vi "program seq..vi"(6 "IOList":T3, 7 "Cluster data":T5, 11 "Filepath":path=path "E:/My Project/2018-2019/Under development/Minda Ind. Switch -ID 144-145/Project/data/trail pro -12.txt") -> (0 "Error Out":errorcluster)   [LabVIEW 2015]
uses:
  Control PB/Active.ctl
  Control PB/deactive.ctl
  Control PB/output control.ctl
  Control PB/input control.ctl
  Control PB/timer.ctl
  Control PB/Remove list.ctl
  Control Button/Exit.ctl
  Control PB/Add_s.ctl
  Control PB/Delete_.ctl
  Control Button/Save.ctl
  Control PB/motor.ctl
  Control PB/Camera.ctl
  Control PB/Barcode.ctl
  Galobal variable_TI.vi
panel:
  out "Step List 5":string[](array[string])
  in  "CAN":bool
  in  "Feature Step edit":bool
  out "Step List 4":string[](array[string])
  out "Step List 3":string[](array[string])
  in  "Barcode":T1
  in  "Camera":T2
  out "x <= y?":bool
  out "Cancel":bool
  out "Step List 2":string[](array[string])
  out "Pokayoka Result":cluster{"Sensor Name":string, "Boolean":bool}[](array[cluster])
  in  "Feed Back Channel":i32[](listbox)=[0]
  out "Input":bool[](array[boolean])
  out "Feature List (Out) 2":T4(array[cluster])
  out "error out 2":errorcluster
  in  "Control":bool
  out "Station No":string
  out "Model Name":string
  out "Model":string
  in  "Motor":T6
  in  "Feature List":i32(listbox) caption="Steps List"
  in  "Deletefeature list":T7
  in  "Add feature list":T8
  in  "Deactive":T9
  in  "Active":T10
  in  "Program step":i32(listbox)
  in  "Remove Step":T11
  in  "Wait Time":u32=100 caption="Timer(ms)" max=600000 step=1
  in  "Timer":T12
  in  "Save":T13
  in  "stop":T14
  in  "op Add":T15
  in  "Input Add":T16
  out "Step List":string[](array[string])
  out "output cluster":T17
  in  "Analog":bool
  in  "Analog Input":i32[](listbox)=[0]
  in  "Control Channel":i32[](listbox)=[7]
  in  "Steps":T18(array[cluster])
  in  "Program mode":string="Data"
  out "error out":errorcluster
  out "Feature List (Out)":T19(array[cluster])
  # "Program Sequence Window"
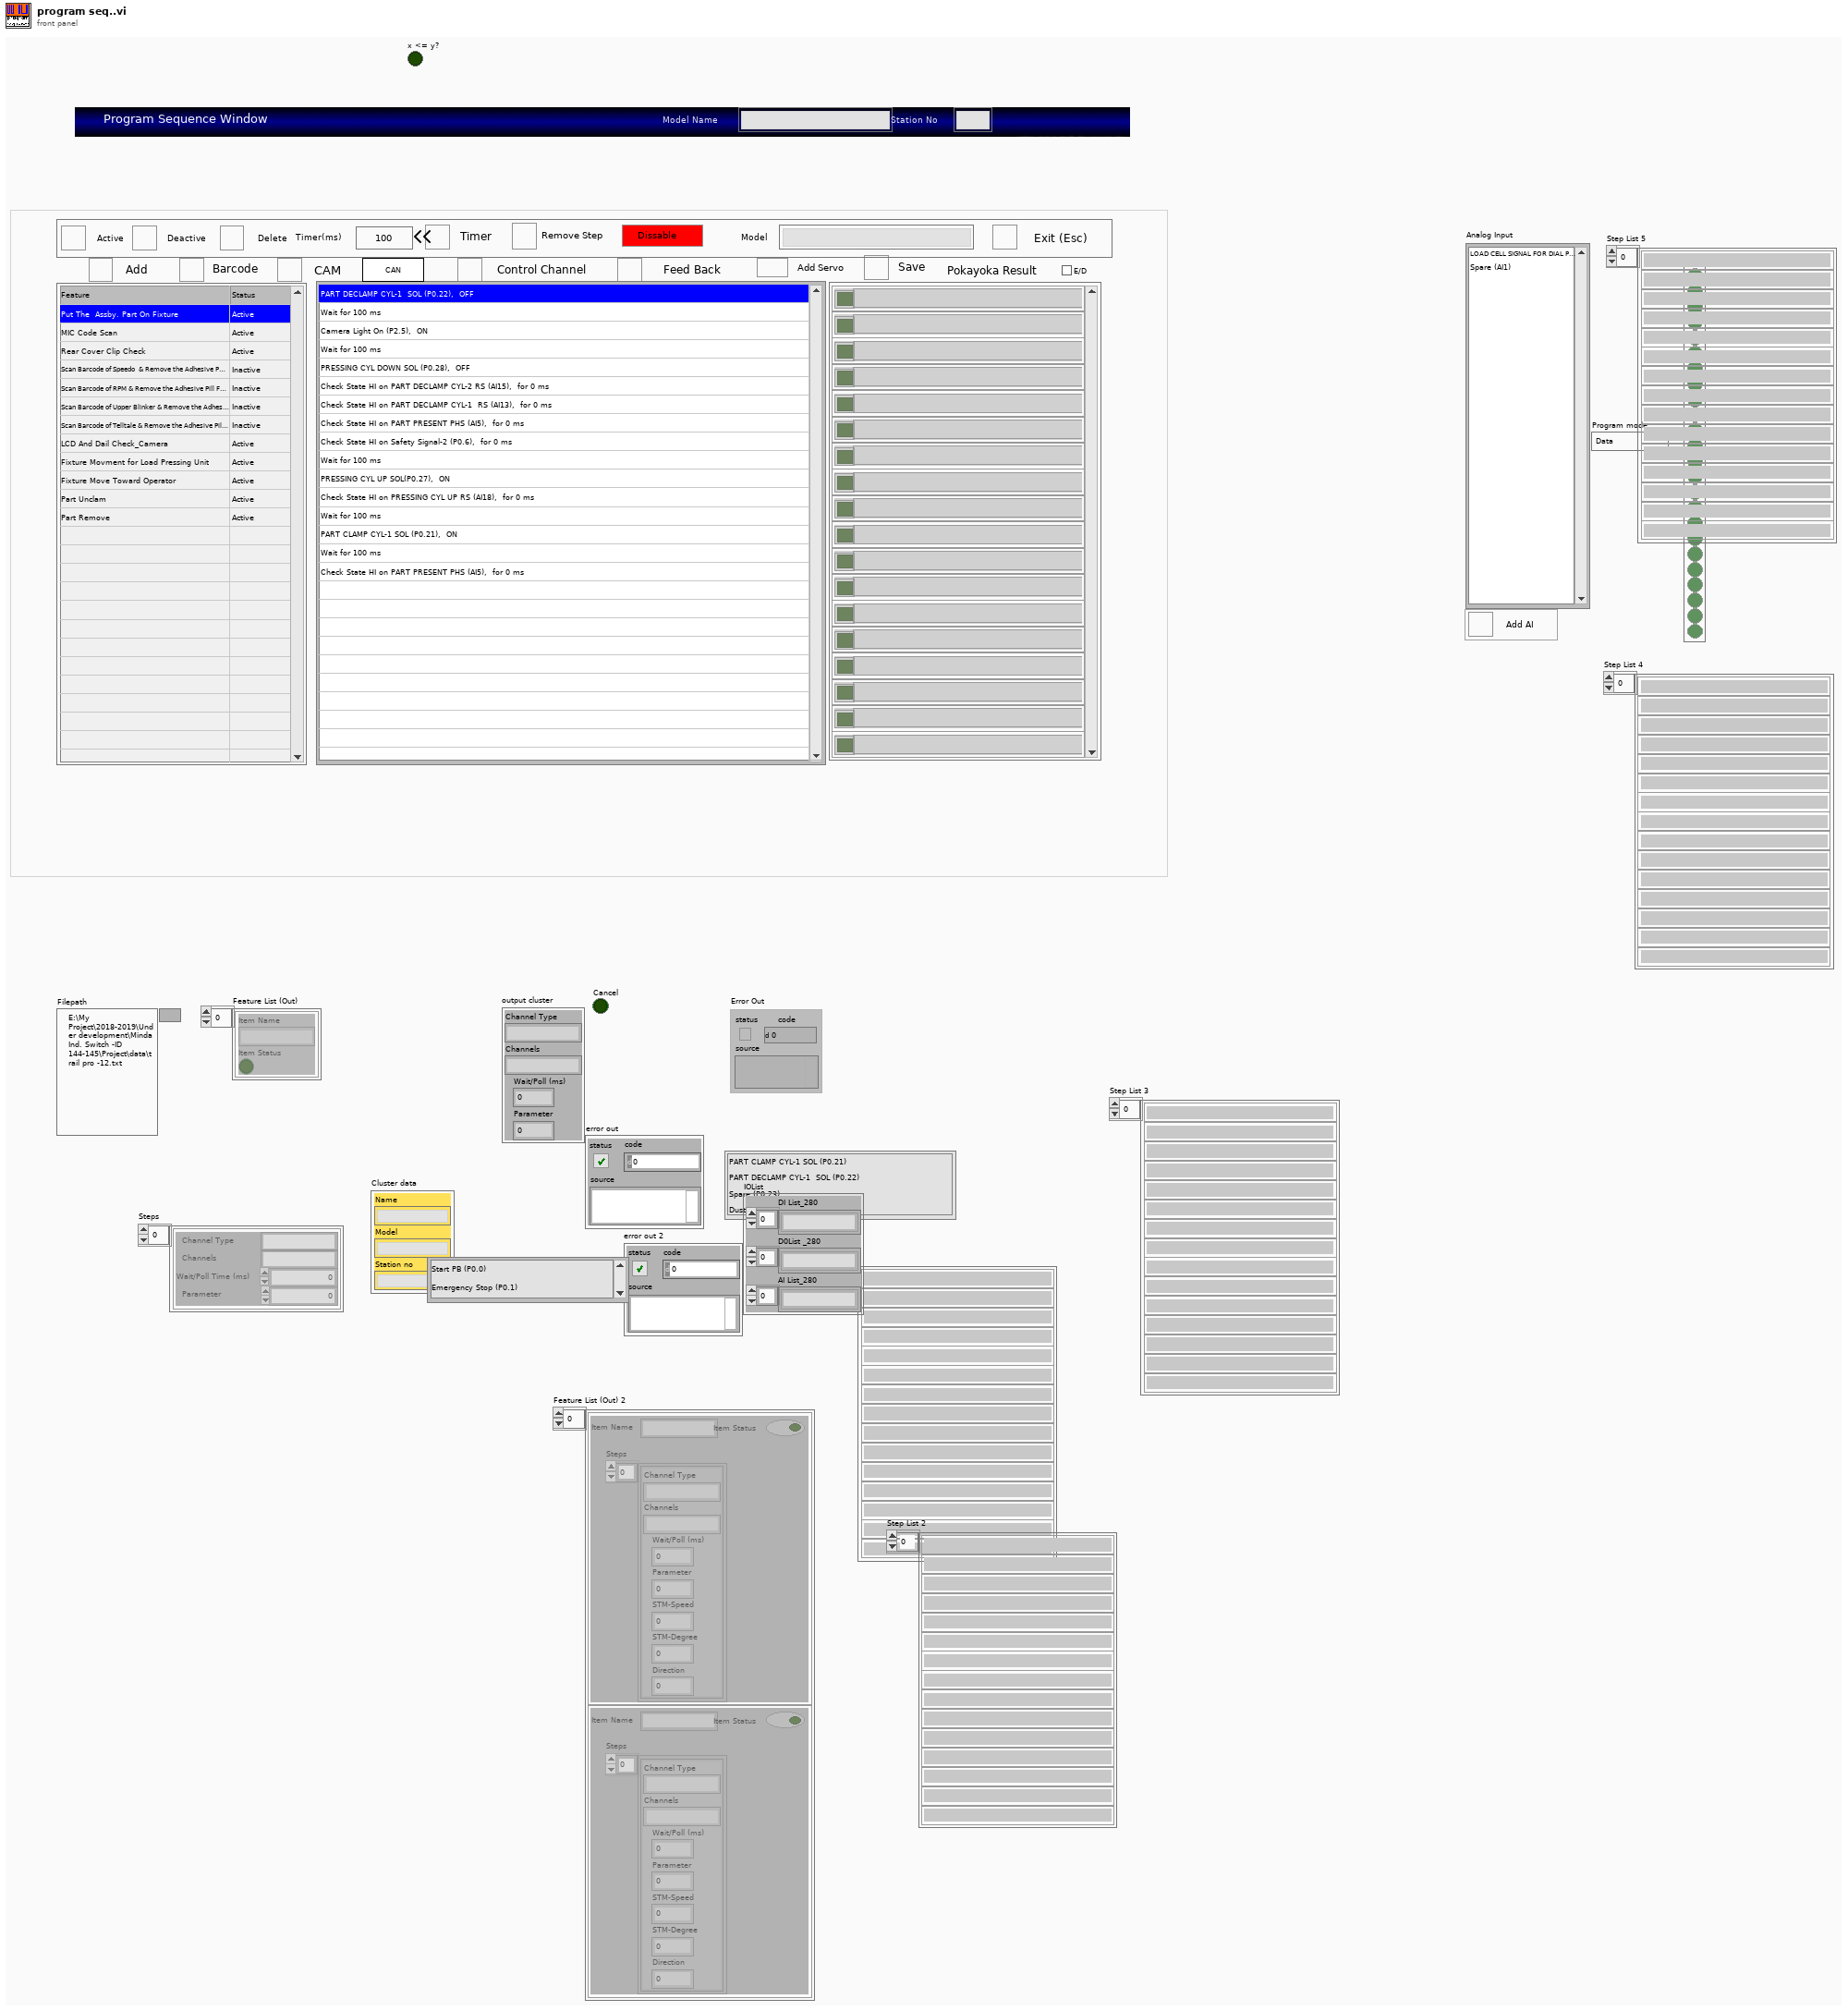
[diagram p1: front panel]
types:
  T1 = typedef "Barcode.ctl" = bool
  T2 = typedef "Camera.ctl" = bool
  T3 = cluster{"DI List_280":string[], "D0List _280":string[], "AI List_280":string[]}
  T4 = cluster{"Item Name":string, "Item Status":bool, "Steps":cluster{"Channel Type":string, "Channels":string, "Wait/Poll (ms)":u32, "Parameter":u8, "STM-Speed":i32, "STM-Degree":u32, "Direction":u8}[]}[]
  T5 = cluster{"Name":string, "Model":string, "Station no":string}
  T6 = typedef "motor.ctl" = bool
  T7 = typedef "Delete_.ctl" = bool
  T8 = typedef "Add_s.ctl" = bool
  T9 = typedef "deactive.ctl" = bool
  T10 = typedef "Active.ctl" = bool
  T11 = typedef "Remove list.ctl" = bool
  T12 = typedef "timer.ctl" = bool
  T13 = typedef "Save.ctl" = bool
  T14 = typedef "Exit.ctl" = bool
  T15 = typedef "output control.ctl" = bool
  T16 = typedef "input control.ctl" = bool
  T17 = cluster{"Channel Type":string, "Channels":string, "Wait/Poll (ms)":u32, "Parameter":u8}
  T18 = cluster{"Channel Type":string, "Channels":string, "Wait/Poll Time (ms)":u32, "Parameter":u8}[]
  T19 = cluster{"Item Name":string, "Item Status":bool}[]
  T20 = cluster{"Channel Type":string, "Channels":string, "Wait/Poll (ms)":u32, "Parameter":u8, "STM-Speed":i32, "STM-Degree":i32, "Direction":u8}
  T21 = cluster{"Item Name":string, "Item Status":bool, "Steps":cluster{"Channel Type":string, "Channels":string, "Wait/Poll (ms)":u32, "Parameter":u8, "STM-Speed":i32, "STM-Degree":u32, "Direction":u8}[]}
  T22 = cluster{"Channel Type":string, "Channels":string, "Wait/Poll (ms)":u32, "Parameter":u8, "STM-Speed":i32, "STM-Degree":u32, "Direction":u8}[]
  T23 = typedef "CAN.ctl" = enum16{"TFT/LCD Power On", "TFT/LCD Power Off", "KM CHeck"}
  T24 = cluster{"Item Name":string, "Active":T10, "Steps":cluster{"Channel Type":string, "Channels":string, "Wait/Poll (ms)":u32, "Parameter":u8, "STM-Speed":i32, "STM-Degree":u32, "Direction":u8}[]}
  T25 = cluster{"Channel Type":string, "Channels":string, "Wait/Poll (ms)":u32, "Parameter":u8, "STM-Speed":i32, "STM-Degree":i32, "Direction":u8}[]
  T26 = cluster{"Feature name ":string, bool, cluster{"Channel Type":string, "Channels":string, "Wait/Poll (ms)":u32, "Parameter":u8, "STM-Speed":i32, "STM-Degree":i32, "Direction":u8}[]}
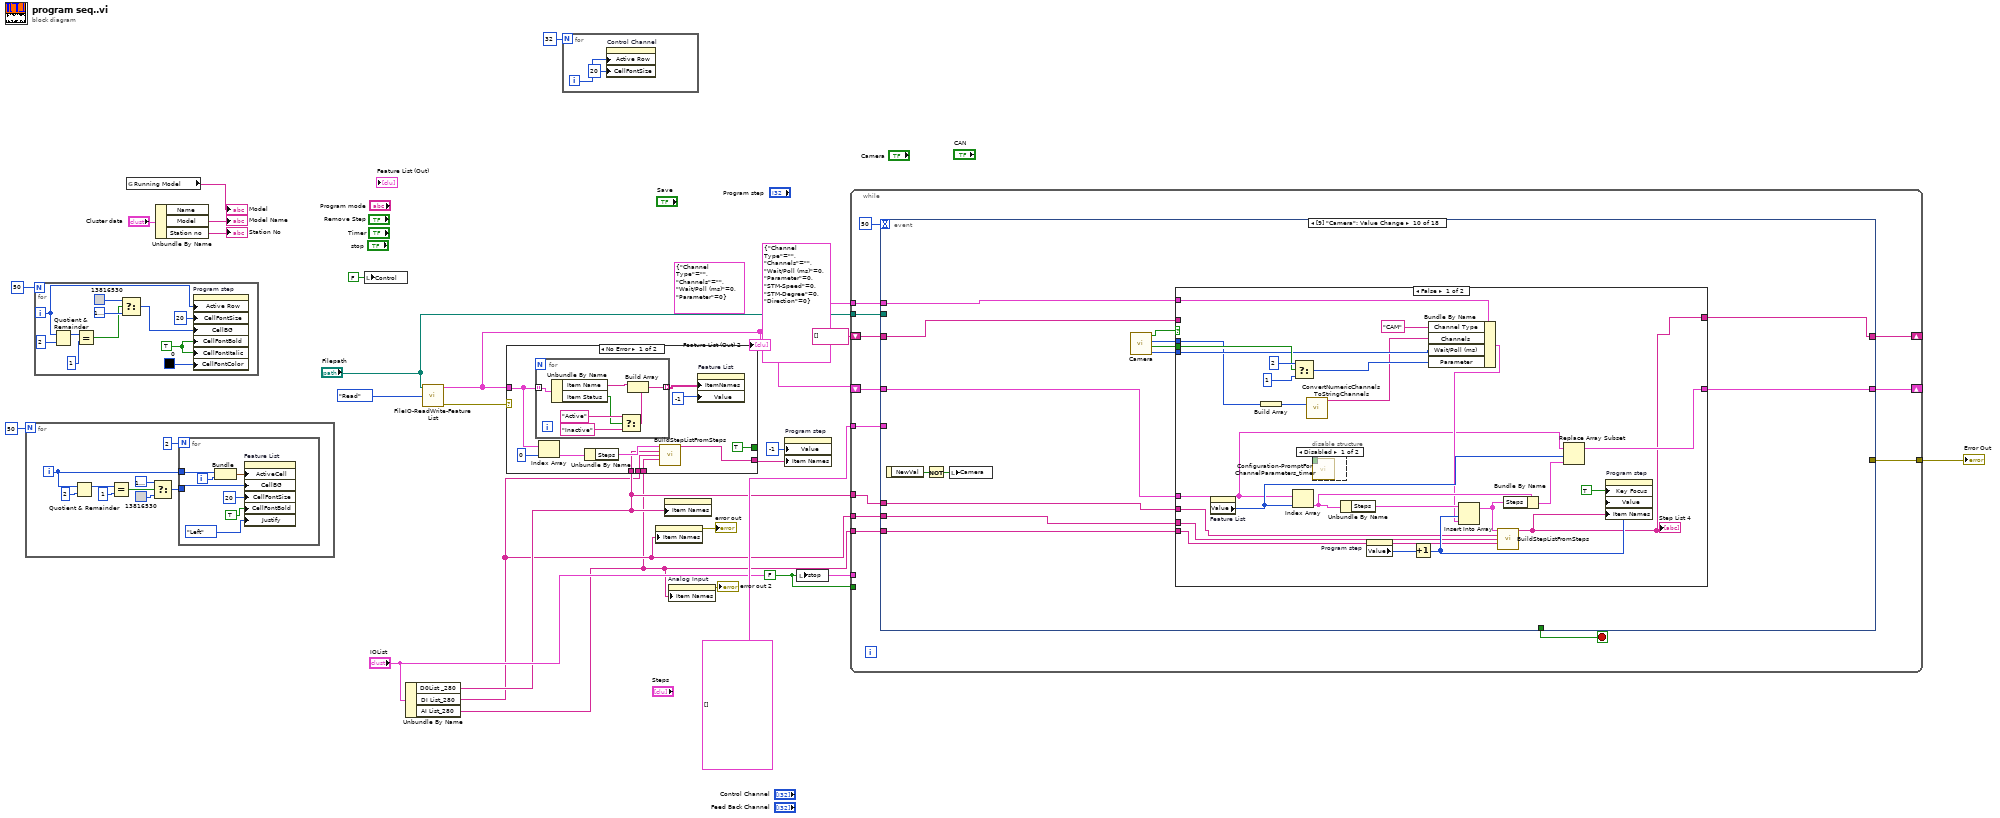
[diagram p0: block diagram]
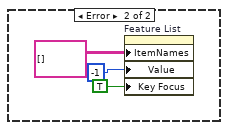
[diagram p2: hidden frame]
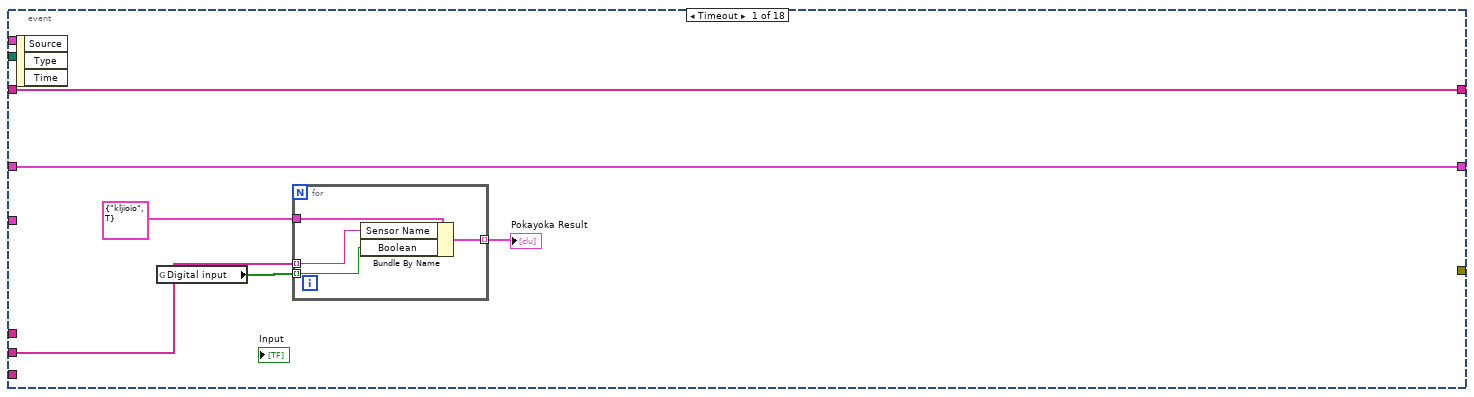
[diagram p3: hidden frame]
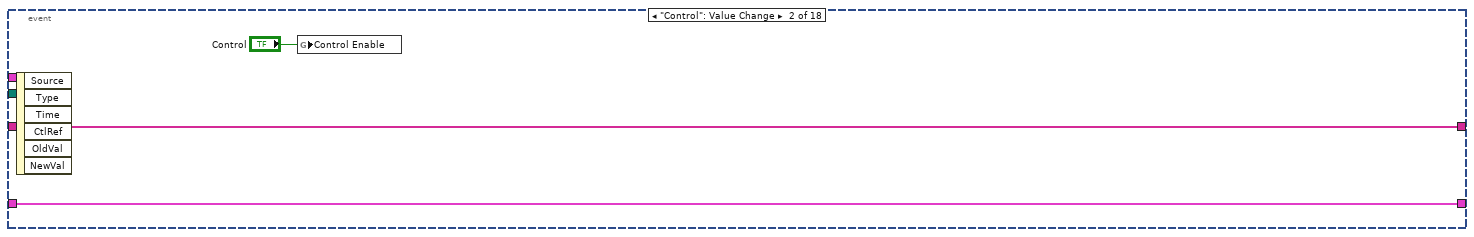
[diagram p4: hidden frame]
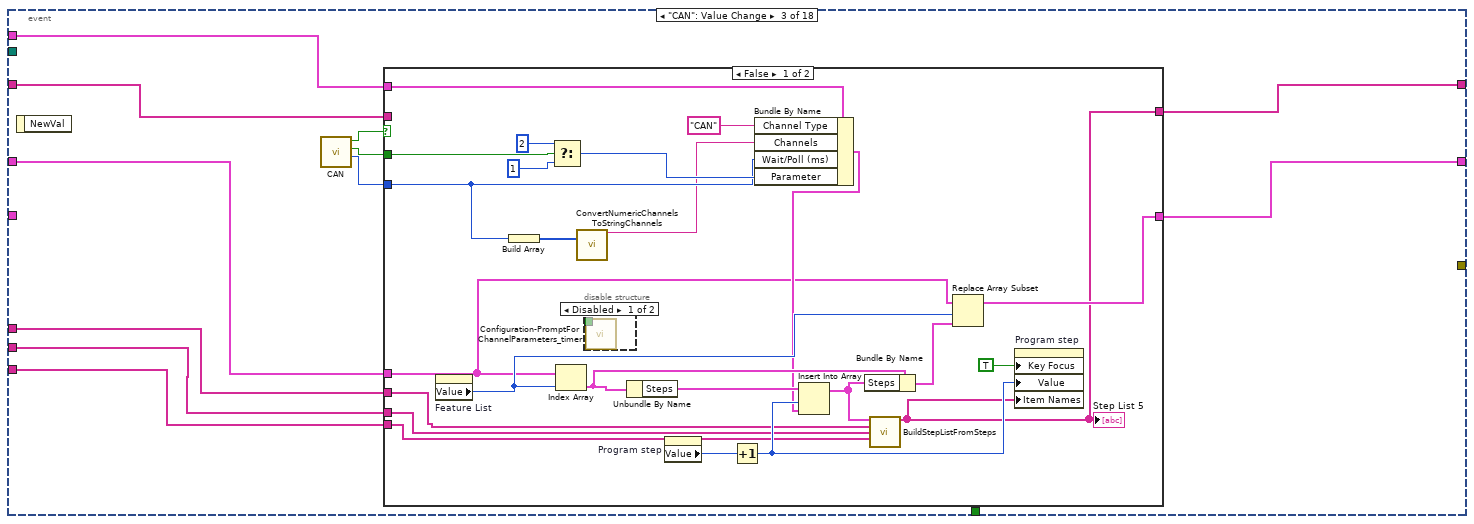
[diagram p5: hidden frame]
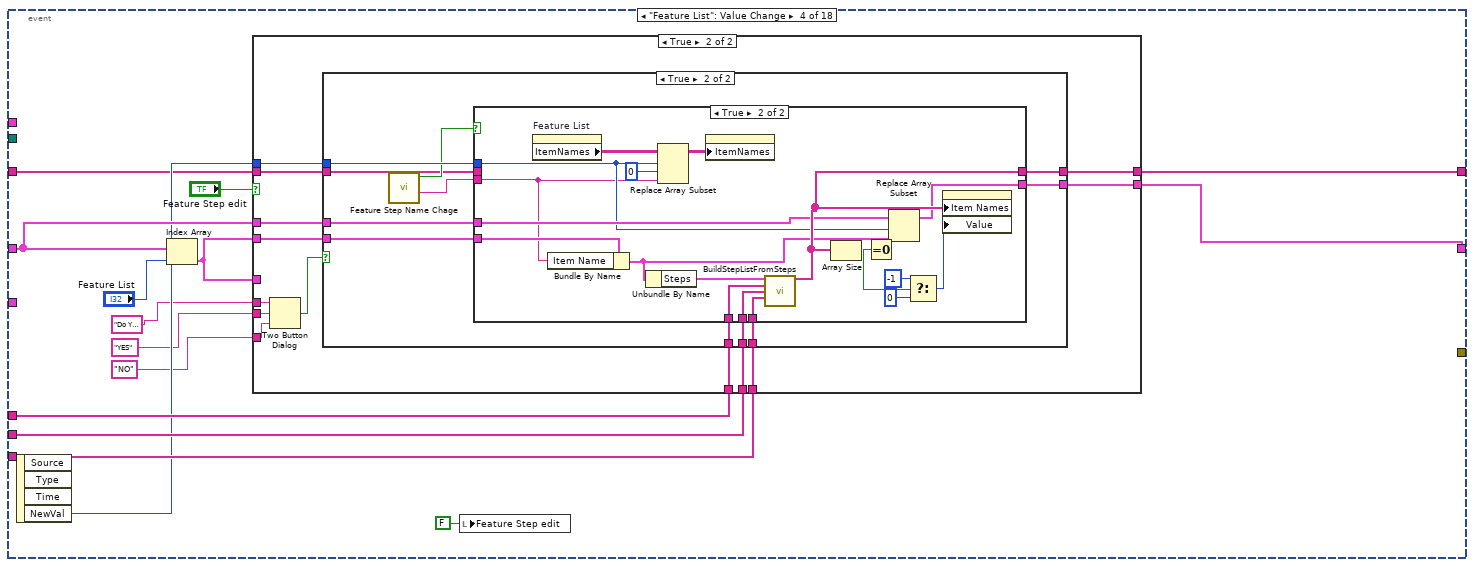
[diagram p8: hidden frame]
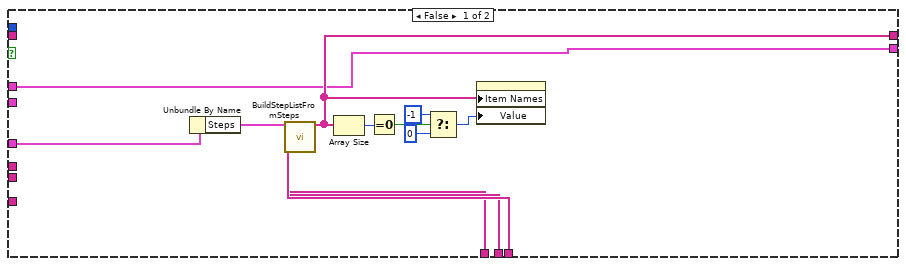
[diagram p9: hidden frame]
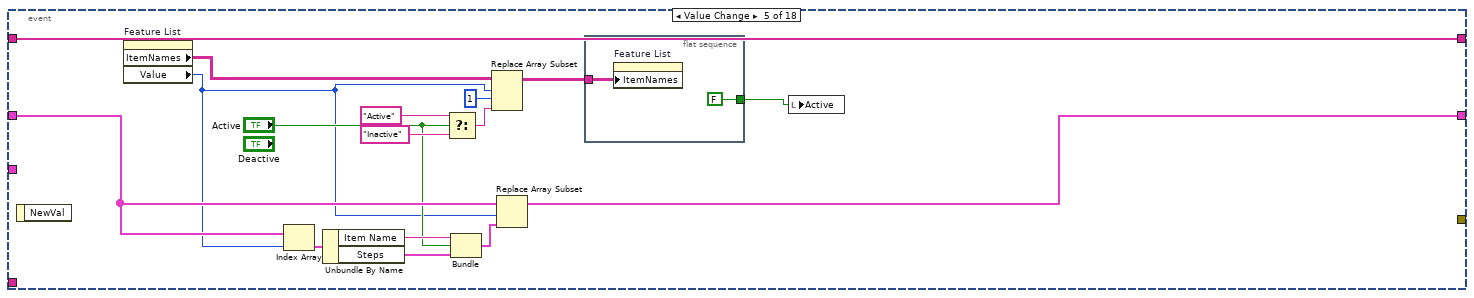
[diagram p12: hidden frame]
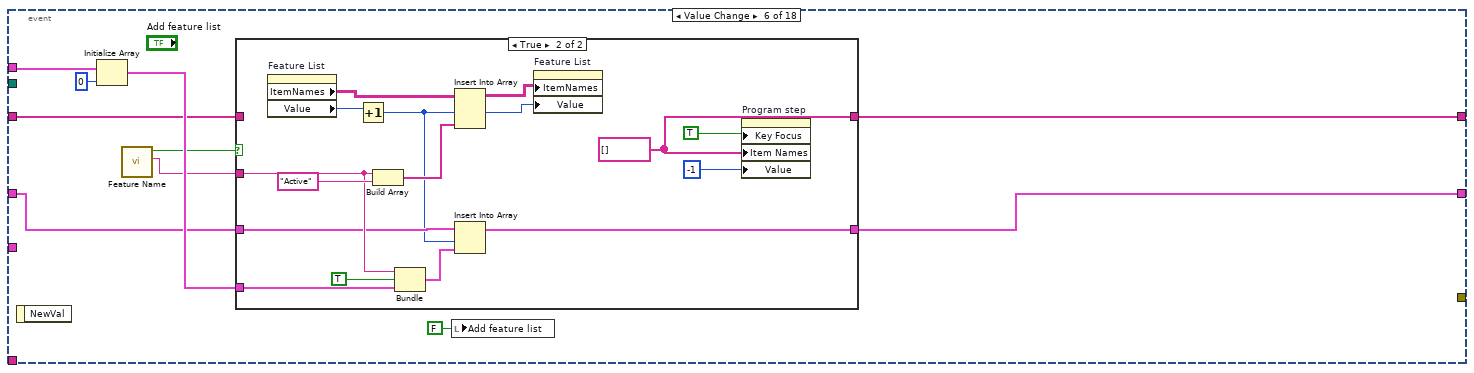
[diagram p13: hidden frame]
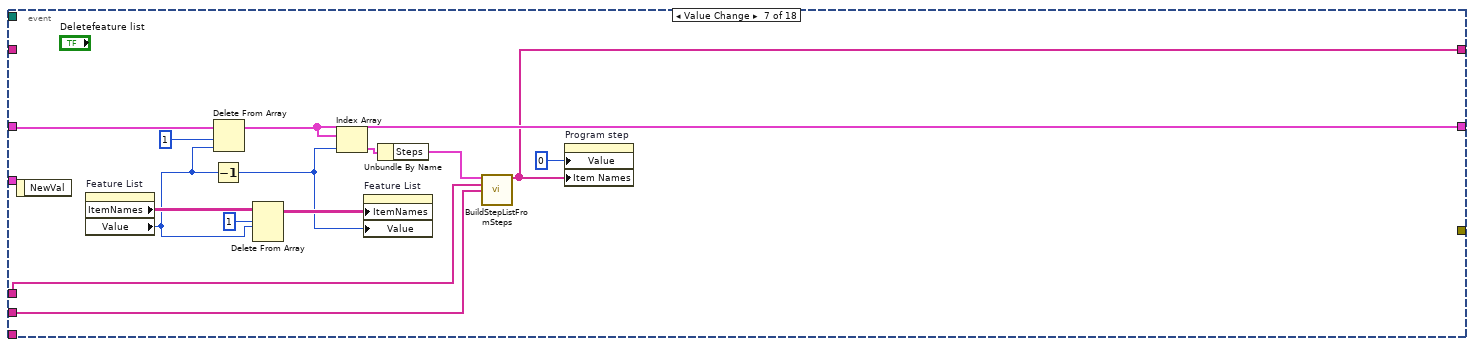
[diagram p15: hidden frame]
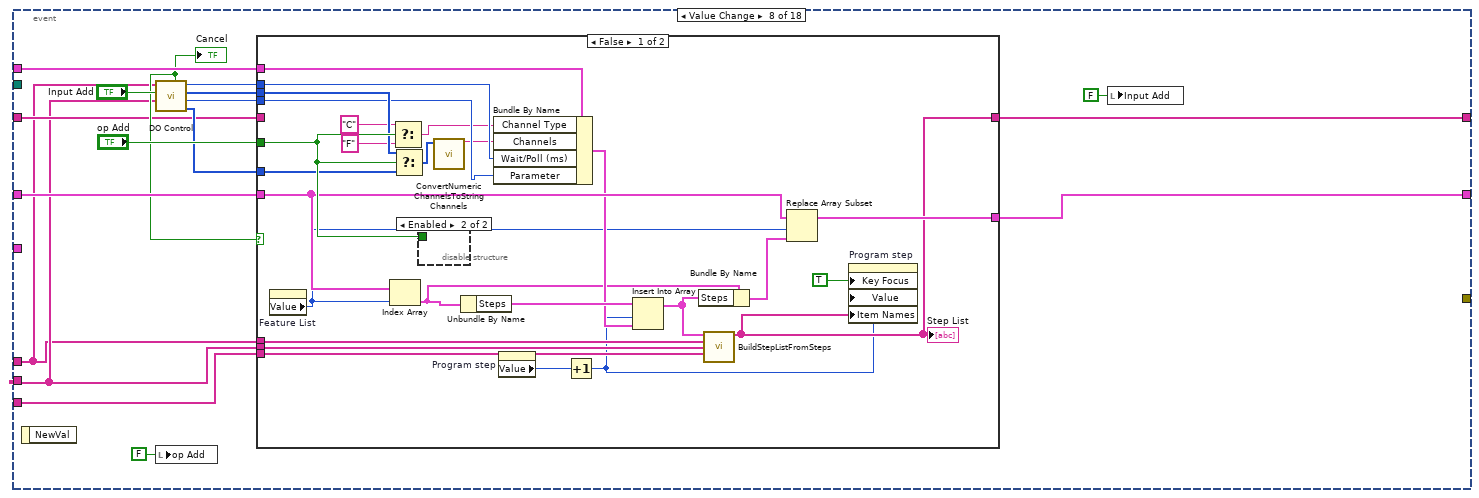
[diagram p16: hidden frame]
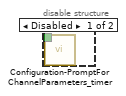
[diagram p17: hidden frame]
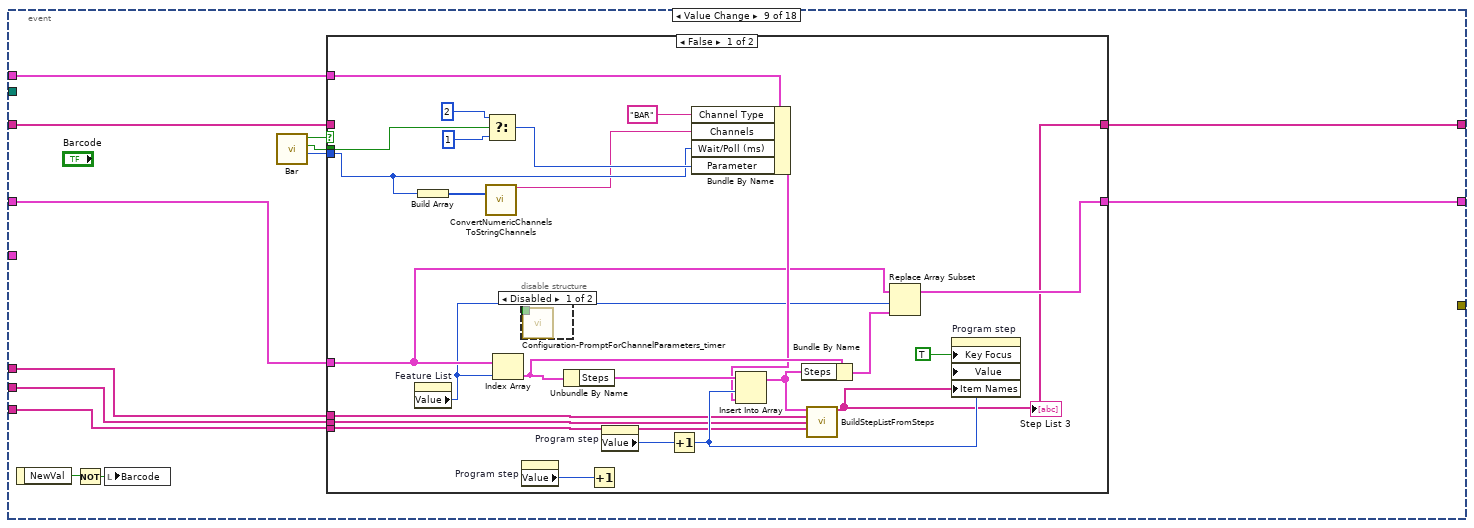
[diagram p19: hidden frame]
diagram:
  w9 = FALSE ("stop")
  (unwired) T17 {"Channel Type"="", "Channels"="", "Wait/Poll (ms)"=0, "Parameter"=0} ("Step")
  n1 = for {
    N: 50 -> [_]
    i -> [w33]
    n2 = Quotient & Remainder(x=w33, y=2) -> (x-y*floor(x/y)=w31:i32)  [unwired: 1 out]
    n3 = Equal?(x=w31, y=1) -> (x = y?=w29:bool)
    n4 = Select(t=u32 16777225 ("Color Box"), s=w29, f=u32 13816530 ("Color Box")) -> (s? t:f=w26:u32)
    n5 = for {
      N: 2 -> [_]
      tunnel: w33 -> [w41]
      tunnel: w26 -> [w38]
      i -> [w40]
      n6 = Bundle(w41, w40) -> (w39:cluster{i32, i32})  [unwired: 1 in]
      n7 = property on="Feature List" class="MCListbox (strict)"("ActiveCell"=w39, "CellBG"=w38, "CellFontSize"=u32 20 ("Active Cell:Cell Font:Size"), "CellFontBold"=TRUE ("Active Cell:Cell Font:Bold"), "Justify"=enum16{"Left", "Center", "Right"}."Left" ("Active Cell:Cell Justification")) -> ()  [unwired: 2 in, 2 out]
    }
  }
  n8 = for {
    N: 50 -> [_]
    i -> [w46]
    w43 = TRUE
    n9 = Quotient & Remainder(x=w46, y=2) -> (x-y*floor(x/y)=w49:i32)  [unwired: 1 out]
    n10 = Equal?(x=w49, y=1) -> (x = y?=w47:bool)
    n11 = Select(t=u32 13816530 ("Color Box"), s=w47, f=u32 16777226 ("Color Box")) -> (s? t:f=w44:u32)
    n12 = property on="Program step" class="LstBox (strict)"("Active Row"=w46, "CellFontSize"=u32 20 ("Active Row:Cell Font:Size"), "CellBG"=w44, "CellFontBold"=w43, "CellFontItalic"=w43, "CellFontColor"=u32 0 ("Color Box")) -> ()  [unwired: 2 in, 2 out]
  }
  n13 = global read "Galobal variable_TI.vi" "Running Model"() -> (→"Model":string)
  n14 = Unbundle By Name("Cluster data") -> ("Model"=→"Model Name":string, "Station no"=→"Station No":string)  [unwired: 1 out]
  n15 = local write "Control"(FALSE ("Control")) -> ()
  n16 = Unbundle By Name("IOList") -> ("D0List _280"=w5:string[], "DI List_280"=w4:string[], "AI List_280"=w3:string[])
  n17 = call "FileIO-ReadWrite-FeatureList.vi"("Filepath"="Filepath", "Read/Write"=enum16{"Read", "Write"}."Read") -> ("Feature List (Out)"=w16:T4, "Error Out"=w20:errorcluster)  [unwired: 12 in]
  "Feature List (Out) 2" <- w16
  n18 = case shown="No Error" w20 {
    tunnel: w16 -> [w63 _]
    tunnel: w5 -> [w59 _]
    tunnel: w4 -> [w58 _]
    tunnel: w3 -> [w57 _]
    tunnel: [w56 _] -> w19
    tunnel: [TRUE ("Key Focus") _] -> _
    frame No Error {
      n19 = for {
        tunnel: w63 -> [w70] mode=indexing
        tunnel: [w64] -> w54 mode=indexing
        n20 = Unbundle By Name(w70) -> ("Item Name"=w66:string, "Item Status"=w67:bool)
        n21 = Select(t="Active", s=w67, f="Inactive") -> (s? t:f=w65:string)
        n22 = Build Array(w66, w65) -> (w64:string[])
      }
      n23 = Index Array(array=w63, index=0) -> (element=w61:T21)
      n24 = Unbundle By Name(w61) -> ("Steps"=w60:T22)
      n25 = call "BuildStepListFromSteps.vi"("Steps"=w60, "Control Channels"=w59, "Feedback Channels"=w58, "AI"=w57) -> ("Step List"=w56:string[])  [unwired: 11 in]
      n26 = property on="Feature List" class="MCListbox (strict)"("ItemNames"=w54, "Value"=-1 ("Feautre list")) -> ()  [unwired: 2 in, 2 out]
    }
    frame Error {
      n27 = property on="Feature List" class="MCListbox (strict)"("ItemNames"=string[][] [] ("Item Names"), "Value"=-1 ("Feautre list"), "Key Focus"=TRUE) -> ()  [unwired: 2 in, 2 out]
    }
  }
  n28 = for {
    N: 32 -> [_]
    i -> [w75]
    n29 = property on="Control Channel" class="LstBox (strict)"("Active Row"=w75, "CellFontSize"=u32 20 ("Active Row:Cell Font:Size")) -> ()  [unwired: 2 in, 2 out]
  }
  n30 = property on="Feed Back Channel" class="LstBox (strict)"("Item Names"=w4) -> (error out=→"error out":errorcluster)  [unwired: 2 in, 1 out]
  n31 = property on="Control Channel" class="LstBox (strict)"("Item Names"=w5) -> ()  [unwired: 2 in, 2 out]
  n32 = property on="Analog Input" class="LstBox (strict)"("Item Names"=w3) -> (error out=→"error out 2":errorcluster)  [unwired: 2 in, 1 out]
  n33 = property on="Program step" class="LstBox (strict)"("Value"=-1 ("Step feautre list"), "Item Names"=w19) -> ()  [unwired: 2 in, 2 out]
  n34 = local write "stop"(w9) -> ()
  n35 = while {
    shift-right: [w86] -> _
    shift-left: w16 -> [w77]
    tunnel: T20 {"Channel Type"="", "Channels"="", "Wait/Poll (ms)"=0, "Parameter"=0, "STM-Speed"=0, "STM-Degree"=0, "Direction"=0} ("Step") -> [w87]
    shift-right: [w85] -> _
    shift-left: string[] [] ("Step List") -> [w84]
    tunnel: w5 -> [w83]
    tunnel: w4 -> [w82]
    tunnel: [w81] -> w23
    tunnel: w3 -> [w80]
    tunnel: T4 [] ("Feature List (Out) 2") -> [w79]
    tunnel: "Filepath" -> [w78]
    tunnel: w9 -> [_]
    tunnel: "IOList" -> [_]
    stop <- w88 stop-if-true
    n36 = event shown="[9] \"Camera\": Value Change" {
      selector: _ -> [_ _ _ _ _ _ _ _ _ _ _ _ _ _ _ _ _ _]
      dyn-events: _ -> [_ _ _ _ _ _ _ _ _ _ _ _ _ _ _ _ _ _]
      timeout: 50 -> [_ _ _ _ _ _ _ _ _ _ _ _ _ _ _ _ _ _]
      tunnel: [_ _ _ _ _ _ _ _ _ _ _ _ _ _ _ TRUE ("stop") _ TRUE ("Discard?")] -> w88
      tunnel: w77 -> [w94 w100 w102 w148 w221 w238 w270 w286 w326 w369 w411 w441 w462 w484 w493 w553 w575 w652]
      tunnel: w87 -> [_ _ w109 _ _ w241 _ w289 w331 w373 w418 w446 w471 _ _ _ w576 _]
      tunnel: [w94 w100 w103 w147 w219 w237 w269 w287 w325 w368 w406 w433 w461 w483 w495 w553 w571 w652] -> w86
      tunnel: [w93 w101 w107 w154 w218 w234 w264 w285 w324 w367 w405 w432 w458 w478 w510 w552 w570 w653] -> w85
      tunnel: w84 -> [w93 w101 w108 w140 w218 w233 _ w276 w319 w363 _ _ _ _ _ w552 w569 w653]
      tunnel: w83 -> [_ _ w112 w153 _ _ w266 w274 w327 w370 w408 w438 w460 w480 w512 _ w572 _]
      tunnel: w82 -> [w92 _ w111 w152 _ _ w265 w275 w328 w371 w409 w437 w459 w479 w511 _ w573 _]
      tunnel: [_ _ _ _ _ _ _ _ _ _ _ _ _ _ w503 _ _ _] -> w81
      tunnel: w80 -> [_ _ w110 w151 _ _ _ w284 w329 w372 w410 w436 w457 _ w504 _ w574 _]
      tunnel: w79 -> [_ _ _ _ _ _ _ _ _ _ _ _ _ _ w509 _ _ _]
      tunnel: w78 -> [_ _ _ _ _ _ _ _ _ _ _ _ _ _ w494 _ _ _]
      event Timeout {
        n37 = event-data() -> ()  [unwired: 1 in, 3 out]
        n38 = global read "Galobal variable_TI.vi" "Digital input"() -> (w89:bool[])
        n39 = for {
          tunnel: w92 -> [w97] mode=indexing
          tunnel: cluster{"Sensor Name":string, "Boolean":bool} {"Sensor Name"="kljioio", "Boolean"=TRUE} ("Cluster") -> [w98]
          tunnel: [w96] -> w90 mode=indexing
          tunnel: w89 -> [w95] mode=indexing
          n40 = Bundle By Name(cluster=w98, "Sensor Name"=w97, "Boolean"=w95) -> (w96:cluster{"Sensor Name":string, "Boolean":bool})
        }
        "Pokayoka Result" <- w90
      }
      event "Control": Value Change {
        n41 = event-data() -> ()  [unwired: 1 in, 6 out]
        n42 = global write "Galobal variable_TI.vi" "Control Enable"("Control") -> ()
      }
      event "CAN": Value Change {
        n43 = event-data() -> ()  [unwired: 1 in, 1 out]
        n44 = call "CAN.vi"() -> ("CAN Sele"=w106:T23, "CAN"=w105:bool, "Out"=w104:bool)  [unwired: 9 in]
        n45 = case shown="False" w104 {
          tunnel: w110 -> [w123 _]
          tunnel: w111 -> [w122 _]
          tunnel: w112 -> [w121 _]
          tunnel: w102 -> [w120 w139]
          tunnel: [w119 w139] -> w103
          tunnel: [w118 w138] -> w107
          tunnel: w106 -> [w115 _]
          tunnel: w105 -> [w117 _]
          tunnel: w109 -> [w113 _]
          tunnel: w108 -> [_ w138]
          frame False {
            n46 = property on="Feature List" class="MCListbox (strict)"() -> ("Value"=w125:i32)  [unwired: 2 in, 2 out]
            n47 = Build Array(w115) -> (w116:T23[])
            n48 = Select(t=2, s=w117, f=1) -> (s? t:f=w133:i32)
            n49 = Index Array(array=w120, index=w125) -> (element=w131:T21)
            n50 = call "ConvertNumericChannelsToStringChannels.vi"("Channels (In)"=w116) -> ("Channels (A:B:C:D...) (Out)"=w114:string)  [unwired: 14 in]
            n51 = disable-structure shown="Disabled" {
              disable-tunnel: _ -> [w137 _]
              frame Disabled {
                n52 = call "Configuration-PromptForChannelParameters_timer.vi"("Control/Feedback\n(Default: False = Feedback)"=w137) -> ()  [unwired: 13 in, 2 out]
              }
              frame Enabled {
              }
            }
            n53 = Unbundle By Name(w131) -> ("Steps"=w132:T22)
            n54 = property on="Program step" class="LstBox (strict)"() -> ("Value"=w126:i32)  [unwired: 2 in, 2 out]
            n55 = Increment(x=w126) -> (x+1=w127:i32)
            n56 = Bundle By Name(cluster=w113, "Channel Type"="CAN", "Channels"=w114, "Wait/Poll (ms)"=w115, "Parameter"=w133) -> (w124:T20)
            n57 = Insert Into Array "Insert Into Array"(array=w132, index=w127, new element=w124) -> (w129:T22)
            n58 = Bundle By Name(cluster=w131, "Steps"=w129) -> (w130:T21)
            n59 = call "BuildStepListFromSteps.vi"("Steps"=w129, "Control Channels"=w121, "Feedback Channels"=w122, "AI"=w123) -> ("Step List"=w118:string[])  [unwired: 11 in]
            "Step List 5" <- w118
            n60 = Replace Array Subset(array=w120, new element=w130, index=w125) -> (w119:T4)
            n61 = property on="Program step" class="LstBox (strict)"("Key Focus"=TRUE, "Value"=w127, "Item Names"=w118) -> ()  [unwired: 2 in, 2 out]
          }
          frame True {
          }
        }
      }
      event "Feature List": Value Change {
        n62 = event-data() -> ("NewVal"=w146:i32)  [unwired: 1 in, 3 out]
        n63 = Index Array(array=w148, index="Feature List") -> (element=w145:T21)
        n64 = case shown="True" "Feature Step edit" {
          tunnel: w145 -> [w162 _]
          tunnel: [w156 w176] -> w154
          tunnel: w153 -> [w159 w177]
          tunnel: w152 -> [w160 w179]
          tunnel: w151 -> [w161 w178]
          tunnel: w148 -> [w155 w175]
          tunnel: [w155 w172] -> w147
          tunnel: w146 -> [_ w174]
          tunnel: w145 -> [_ w173]
          tunnel: "Do You Want Change The Feature List Name?" -> [_ w170]
          tunnel: "YES" -> [_ w169]
          tunnel: "NO" -> [_ w168]
          tunnel: w140 -> [_ w167]
          frame False {
            n65 = Unbundle By Name(w162) -> ("Steps"=w166:T22)
            n66 = call "BuildStepListFromSteps.vi"("Steps"=w166, "Control Channels"=w159, "Feedback Channels"=w160, "AI"=w161) -> ("Step List"=w156:string[])  [unwired: 11 in]
            n67 = Array Size(array=w156) -> (size(s)=w164:i32)
            n68 = Equal To 0?(x=w164) -> (x = 0?=w165:bool)
            n69 = Select(t=-1 ("Step List"), s=w165, f=0 ("Step List")) -> (s? t:f=w157:i32)
            n70 = property on="Program step" class="LstBox (strict)"("Item Names"=w156, "Value"=w157) -> ()  [unwired: 2 in, 2 out]
          }
          frame True {
            n71 = Two Button Dialog(message=w170, 1:w168, 2:w169) -> (T button?=w171:bool)
            n72 = case shown="True" w171 {
              tunnel: w179 -> [_ w192]
              tunnel: w178 -> [_ w191]
              tunnel: w177 -> [_ w190]
              tunnel: [w180 w189] -> w176
              tunnel: w175 -> [w181 w188]
              tunnel: w174 -> [_ w187]
              tunnel: w173 -> [_ w186]
              tunnel: [w181 w185] -> w172
              tunnel: w167 -> [w180 w182]
              frame False {
              }
              frame True {
                n73 = call "Feature Step Name Chage.vi"() -> ("Feature Step Nameout"=w184:string, "Next"=w183:bool)  [unwired: 10 in]
                n74 = case shown="True" w183 {
                  tunnel: w192 -> [_ w209]
                  tunnel: w191 -> [_ w208]
                  tunnel: w190 -> [_ w206]
                  tunnel: [w194 w205] -> w189
                  tunnel: w188 -> [w193 w201]
                  tunnel: w187 -> [_ w199]
                  tunnel: w186 -> [_ w198]
                  tunnel: [w193 w196] -> w185
                  tunnel: w184 -> [_ w195]
                  tunnel: w182 -> [w194 _]
                  frame False {
                  }
                  frame True {
                    n75 = property on="Feature List" class="MCListbox (strict)"() -> ("ItemNames"=w204:string[][])  [unwired: 2 in, 2 out]
                    n76 = Bundle By Name(cluster=w198, "Item Name"=w195) -> (w197:T21)
                    n77 = Unbundle By Name(w197) -> ("Steps"=w200:T22)
                    n78 = Replace Array Subset(array=w204, new element=w195, index (row)=w199, index (col)=0 ("disabled index (col)")) -> (w202:string[][])
                    n79 = property on="Feature List" class="MCListbox (strict)"("ItemNames"=w202) -> ()  [unwired: 2 in, 2 out]
                    n80 = call "BuildStepListFromSteps.vi"("Steps"=w200, "Control Channels"=w206, "Feedback Channels"=w209, "AI"=w208) -> ("Step List"=w205:string[])  [unwired: 11 in]
                    n81 = Array Size(array=w205) -> (size(s)=w211:i32)
                    n82 = Equal To 0?(x=w211) -> (x = 0?=w213:bool)
                    n83 = Replace Array Subset(array=w201, new element=w197, index=w199) -> (w196:T4)
                    n84 = Select(t=-1 ("Step List"), s=w213, f=0 ("Step List")) -> (s? t:f=w207:i32)
                    n85 = property on="Program step" class="LstBox (strict)"("Item Names"=w205, "Value"=w207) -> ()  [unwired: 2 in, 2 out]
                  }
                }
              }
            }
          }
        }
        n86 = local write "Feature Step edit"(FALSE ("Feature Step edit")) -> ()
      }
      event Value Change {
        n87 = event-data() -> ()  [unwired: 1 in, 1 out]
        n88 = property on="Feature List" class="MCListbox (strict)"() -> ("ItemNames"=w217:string[][], "Value"=w215:i32)  [unwired: 2 in, 2 out]
        n89 = Index Array(array=w221, index=w215) -> (element=w227:T21)
        n90 = Unbundle By Name(w227) -> ("Item Name"=w228:string, "Steps"=w229:T22)
        n91 = Select(t="Active", s="Active", f="Inactive" ("element")) -> (s? t:f=w224:string)
        n92 = Bundle("Item Name"=w228, "Active"="Active", "Steps"=w229) -> (w226:T24)  [unwired: 1 in]
        n93 = Replace Array Subset(array=w217, new element=w224, index (row)=w215, index (col)=1 ("disabled index (col)")) -> (w216:string[][])
        n94 = Replace Array Subset(array=w221, new element=w226, index=w215) -> (w219:T4)
        n95 = flat-sequence {
          tunnel: w216 -> [w231]
          tunnel: [T10 FALSE ("Active")] -> w214
          frame #0 {
            n96 = property on="Feature List" class="MCListbox (strict)"("ItemNames"=w231) -> ()  [unwired: 2 in, 2 out]
          }
        }
        n97 = local write "Active"(w214) -> ()
      }
      event Value Change {
        n98 = event-data() -> ()  [unwired: 1 in, 1 out]
        n99 = Initialize Array(w241, 0 ("dimension size")) -> (w239:T25)
        n100 = call "Feature Name.vi"() -> ("Feature name"=w235:string, "Out"=w236:bool)  [unwired: 10 in]
        n101 = case shown="True" w236 {
          tunnel: w239 -> [_ w257]
          tunnel: w238 -> [w243 w252]
          tunnel: [w243 w254] -> w237
          tunnel: w235 -> [_ w253]
          tunnel: [w242 w250] -> w234
          tunnel: w233 -> [w242 _]
          frame False {
          }
          frame True {
            w250 = string[] [] ("Item Names")
            n102 = property on="Feature List" class="MCListbox (strict)"() -> ("ItemNames"=w247:string[][], "Value"=w244:i32)  [unwired: 2 in, 2 out]
            n103 = Increment(x=w244) -> (x+1=w245:i32)
            n104 = Build Array(w253, "Active") -> (w248:string[])
            n105 = Bundle("Feature name"=w253, TRUE, w257) -> (w255:T26)  [unwired: 1 in]
            n106 = Insert Into Array(array=w247, index (row)=w245, new element=w248) -> (w246:string[][])  [unwired: 1 in]
            n107 = Insert Into Array(array=w252, index=w245, new element=w255) -> (w254:T4)
            n108 = property on="Feature List" class="MCListbox (strict)"("ItemNames"=w246, "Value"=w245) -> ()  [unwired: 2 in, 2 out]
            n109 = property on="Program step" class="LstBox (strict)"("Key Focus"=TRUE, "Item Names"=w250, "Value"=-1 ("Step feautre list")) -> ()  [unwired: 2 in, 2 out]
          }
        }
        n110 = local write "Add feature list"(FALSE ("Add feature list")) -> ()
      }
      event Value Change {
        n111 = event-data() -> ()  [unwired: 1 in, 1 out]
        n112 = property on="Feature List" class="MCListbox (strict)"() -> ("ItemNames"=w262:string[][], "Value"=w261:i32)  [unwired: 2 in, 2 out]
        n113 = Decrement(x=w261) -> (x-1=w259:i32)
        n114 = Delete From Array(array=w270, length=1, index=w261) -> (array with subset deleted=w269:T4)  [unwired: 1 out]
        n115 = Delete From Array(array=w262, length=1, index (row)=w261) -> (array with subset deleted=w260:string[][])  [unwired: 1 in, 1 out]
        n116 = Index Array(array=w269, index=w259) -> (element=w268:T21)
        n117 = property on="Feature List" class="MCListbox (strict)"("ItemNames"=w260, "Value"=w259) -> ()  [unwired: 2 in, 2 out]
        n118 = Unbundle By Name(w268) -> ("Steps"=w267:T22)
        n119 = call "BuildStepListFromSteps.vi"("Steps"=w267, "Control Channels"=w266, "Feedback Channels"=w265) -> ("Step List"=w264:string[])  [unwired: 12 in]
        n120 = property on="Program step" class="LstBox (strict)"("Value"=0 ("Step feautre list"), "Item Names"=w264) -> ()  [unwired: 2 in, 2 out]
      }
      event Value Change {
        n121 = event-data() -> ()  [unwired: 1 in, 1 out]
        n122 = call "DO Control.vi"("DI List_280"=w275, "s"="Input Add", "Control"=w274) -> ("Feedback"=w279:i32[], "Parameter (Out)"=w281:u8, "Control Channel"=w283:i32[], "Poll Time (Out)"=w282:u32, "Cancel"=w277:bool)  [unwired: 3 in, 1 out]
        "Cancel" <- w277
        n123 = local write "op Add"(T15 FALSE ("op Add")) -> ()
        n124 = case shown="False" w277 {
          tunnel: w289 -> [w315 _]
          tunnel: "op Add" -> [w314 _]
          tunnel: [w313 w318] -> w287
          tunnel: w286 -> [w312 w318]
          tunnel: w274 -> [w311 _]
          tunnel: w275 -> [w310 _]
          tunnel: [w309 w317] -> w285
          tunnel: w284 -> [w308 _]
          tunnel: w283 -> [w307 _]
          tunnel: w282 -> [w306 _]
          tunnel: w281 -> [w305 _]
          tunnel: w279 -> [w304 _]
          tunnel: w276 -> [_ w317]
          frame False {
            n125 = property on="Feature List" class="MCListbox (strict)"() -> ("Value"=w290:i32)  [unwired: 2 in, 2 out]
            n126 = Index Array(array=w312, index=w290) -> (element=w296:T21)
            n127 = Select(t="C", s=w314, f="F") -> (s? t:f=w301:string)
            n128 = Select(t=w307, s=w314, f=w304) -> (s? t:f=w300:i32[])
            n129 = disable-structure shown="Enabled" {
              disable-tunnel: w314 -> [w316 _]
              frame Disabled {
                n130 = call "Configuration-PromptForChannelParameters_timer.vi"("Control/Feedback\n(Default: False = Feedback)"=w316) -> ()  [unwired: 13 in, 2 out]
              }
              frame Enabled {
              }
            }
            n131 = call "ConvertNumericChannelsToStringChannels.vi"("Channels (In)"=w300) -> ("Channels (A:B:C:D...) (Out)"=w299:string)  [unwired: 14 in]
            n132 = Unbundle By Name(w296) -> ("Steps"=w298:T22)
            n133 = Bundle By Name(cluster=w315, "Channel Type"=w301, "Channels"=w299, "Wait/Poll (ms)"=w306, "Parameter"=w305) -> (w297:T20)
            n134 = property on="Program step" class="LstBox (strict)"() -> ("Value"=w291:i32)  [unwired: 2 in, 2 out]
            n135 = Increment(x=w291) -> (x+1=w292:i32)
            n136 = Insert Into Array "Insert Into Array"(array=w298, index=w292, new element=w297) -> (w294:T22)
            n137 = Bundle By Name(cluster=w296, "Steps"=w294) -> (w295:T21)
            n138 = call "BuildStepListFromSteps.vi"("Steps"=w294, "Control Channels"=w311, "Feedback Channels"=w310, "AI"=w308) -> ("Step List"=w309:string[])  [unwired: 11 in]
            "Step List" <- w309
            n139 = Replace Array Subset(array=w312, new element=w295, index=w290) -> (w313:T4)
            n140 = property on="Program step" class="LstBox (strict)"("Key Focus"=TRUE, "Value"=w292, "Item Names"=w309) -> ()  [unwired: 2 in, 2 out]
          }
          frame True {
          }
        }
        n141 = local write "Input Add"(T16 FALSE ("Input Add")) -> ()
      }
      event Value Change {
        n142 = event-data() -> ("NewVal"=w322:T1)  [unwired: 1 in]
        n143 = Not(x=w322) -> (.not. x?=w321:T1)
        n144 = local write "Barcode"(w321) -> ()
        n145 = call "Bar.vi"() -> ("Time Out Value"=w323:u8, "Barcode Scane"=w330:bool, "Out"=w320:bool)  [unwired: 9 in]
        n146 = case shown="False" w320 {
          tunnel: w331 -> [w356 _]
          tunnel: w330 -> [w354 _]
          tunnel: w329 -> [w341 _]
          tunnel: w328 -> [w340 _]
          tunnel: w327 -> [w339 _]
          tunnel: w326 -> [w338 w358]
          tunnel: [w337 w358] -> w325
          tunnel: [w336 w359] -> w324
          tunnel: w323 -> [w334 _]
          tunnel: w319 -> [_ w359]
          frame False {
            n147 = property on="Feature List" class="MCListbox (strict)"() -> ("Value"=w335:i32)  [unwired: 2 in, 2 out]
            n148 = Build Array(w334) -> (w333:u8[])
            n149 = call "ConvertNumericChannelsToStringChannels.vi"("Channels (In)"=w333) -> ("Channels (A:B:C:D...) (Out)"=w332:string)  [unwired: 14 in]
            n150 = Select(t=2, s=w354, f=1) -> (s? t:f=w351:i32)
            n151 = Index Array(array=w338, index=w335) -> (element=w349:T21)
            n152 = disable-structure shown="Disabled" {
              disable-tunnel: _ -> [w357 _]
              frame Disabled {
                n153 = call "Configuration-PromptForChannelParameters_timer.vi"("Control/Feedback\n(Default: False = Feedback)"=w357) -> ()  [unwired: 13 in, 2 out]
              }
              frame Enabled {
              }
            }
            n154 = property on="Program step" class="LstBox (strict)"() -> ("Value"=w343:i32)  [unwired: 2 in, 2 out]
            n155 = Unbundle By Name(w349) -> ("Steps"=w350:T22)
            n156 = Increment(x=w343) -> ()  [unwired: 1 out]
            n157 = property on="Program step" class="LstBox (strict)"() -> ("Value"=w344:i32)  [unwired: 2 in, 2 out]
            n158 = Increment(x=w344) -> (x+1=w345:i32)
            n159 = Bundle By Name(cluster=w356, "Channel Type"="BAR", "Channels"=w332, "Wait/Poll (ms)"=w334, "Parameter"=w351) -> (w342:T20)
            n160 = Insert Into Array "Insert Into Array"(array=w350, index=w345, new element=w342) -> (w347:T22)
            n161 = Bundle By Name(cluster=w349, "Steps"=w347) -> (w348:T21)
            n162 = call "BuildStepListFromSteps.vi"("Steps"=w347, "Control Channels"=w339, "Feedback Channels"=w340, "AI"=w341) -> ("Step List"=w336:string[])  [unwired: 11 in]
            "Step List 3" <- w336
            n163 = Replace Array Subset(array=w338, new element=w348, index=w335) -> (w337:T4)
            n164 = property on="Program step" class="LstBox (strict)"("Key Focus"=TRUE, "Value"=w345, "Item Names"=w336) -> ()  [unwired: 2 in, 2 out]
          }
          frame True {
          }
        }
      }
      event Value Change {
        n165 = event-data() -> ("NewVal"=w360:T2)  [unwired: 1 in]
        n166 = Not(x=w360) -> (.not. x?=w361:T2)
        n167 = local write "Camera"(w361) -> ()
        n168 = call "Camera.vi"() -> ("Time Out (ms) 2"=w365:u8, "Camera 2"=w364:bool, "Feature listout"=w366:u16, "Out"=w362:bool)  [unwired: 8 in]
        n169 = case shown="False" w362 {
          tunnel: w373 -> [w385 _]
          tunnel: w372 -> [w384 _]
          tunnel: w371 -> [w383 _]
          tunnel: w370 -> [w382 _]
          tunnel: w369 -> [w381 w400]
          tunnel: [w380 w400] -> w368
          tunnel: [w379 w401] -> w367
          tunnel: w366 -> [w374 _]
          tunnel: w365 -> [w376 _]
          tunnel: w364 -> [w378 _]
          tunnel: w363 -> [_ w401]
          frame False {
            n170 = property on="Feature List" class="MCListbox (strict)"() -> ("Value"=w387:i32)  [unwired: 2 in, 2 out]
            n171 = Build Array(w374) -> (w377:u16[])
            n172 = Index Array(array=w381, index=w387) -> (element=w393:T21)
            n173 = Select(t=2, s=w378, f=1) -> (s? t:f=w395:i32)
            n174 = call "ConvertNumericChannelsToStringChannels.vi"("Channels (In)"=w377) -> ("Channels (A:B:C:D...) (Out)"=w375:string)  [unwired: 14 in]
            n175 = disable-structure shown="Disabled" {
              disable-tunnel: _ -> [w399 _]
              frame Disabled {
                n176 = call "Configuration-PromptForChannelParameters_timer.vi"("Control/Feedback\n(Default: False = Feedback)"=w399) -> ()  [unwired: 13 in, 2 out]
              }
              frame Enabled {
              }
            }
            n177 = Unbundle By Name(w393) -> ("Steps"=w394:T22)
            n178 = property on="Program step" class="LstBox (strict)"() -> ("Value"=w388:i32)  [unwired: 2 in, 2 out]
            n179 = Increment(x=w388) -> (x+1=w389:i32)
            n180 = Bundle By Name(cluster=w385, "Channel Type"="CAM", "Channels"=w375, "Wait/Poll (ms)"=w376, "Parameter"=w395) -> (w386:T20)
            n181 = Insert Into Array "Insert Into Array"(array=w394, index=w389, new element=w386) -> (w391:T22)
            n182 = call "BuildStepListFromSteps.vi"("Steps"=w391, "Control Channels"=w382, "Feedback Channels"=w383, "AI"=w384) -> ("Step List"=w379:string[])  [unwired: 11 in]
            "Step List 4" <- w379
            n183 = Bundle By Name(cluster=w393, "Steps"=w391) -> (w392:T21)
            n184 = Replace Array Subset(array=w381, new element=w392, index=w387) -> (w380:T4)
            n185 = property on="Program step" class="LstBox (strict)"("Key Focus"=TRUE, "Value"=w389, "Item Names"=w379) -> ()  [unwired: 2 in, 2 out]
          }
          frame True {
          }
        }
      }
      event "Analog": Value Change {
        n186 = event-data() -> ()  [unwired: 1 in, 1 out]
        n187 = property on="Feature List" class="MCListbox (strict)"() -> ("Value"=w402:i32)  [unwired: 2 in, 2 out]
        n188 = call "Configuration-PromptForChannelParameters_timer.vi"("Control/Feedback\n(Default: False = Feedback)"=FALSE ("Control/Feedback\n(Default: False = Feedback)")) -> ("Poll Time (Out)"=w422:u32, "Parameter (Out)"=w421:u8)  [unwired: 13 in]
        n189 = Select(t="AI", s="Analog", f="N") -> (s? t:f=w424:string)
        n190 = call "ConvertNumericChannelsToStringChannels.vi"("Channels (In)"="Analog Input") -> ("Channels (A:B:C:D...) (Out)"=w423:string)  [unwired: 14 in]
        n191 = property on="Program step" class="LstBox (strict)"() -> ("Value"=w412:i32)  [unwired: 2 in, 2 out]
        n192 = Bundle By Name(cluster=w418, "Channel Type"=w424, "Channels"=w423, "Wait/Poll (ms)"=w422, "Parameter"=w421) -> (w407:T20)
        n193 = Index Array(array=w411, index=w402) -> (element=w416:T21)
        n194 = Increment(x=w412) -> (x+1=w403:i32)
        n195 = Unbundle By Name(w416) -> ("Steps"=w417:T22)
        n196 = Insert Into Array(array=w417, index=w403, new element=w407) -> (w414:T22)
        n197 = Bundle By Name(cluster=w416, "Steps"=w414) -> (w415:T21)
        n198 = call "BuildStepListFromSteps.vi"("Steps"=w414, "Control Channels"=w408, "Feedback Channels"=w409, "AI"=w410) -> ("Step List"=w405:string[])  [unwired: 11 in]
        n199 = Replace Array Subset(array=w411, new element=w415, index=w402) -> (w406:T4)
        n200 = property on="Program step" class="LstBox (strict)"("Key Focus"=TRUE, "Value"=w403, "Item Names"=w405) -> ()  [unwired: 2 in, 2 out]
      }
      event Value Change {
        n201 = event-data() -> ()  [unwired: 1 in, 1 out]
        n202 = property on="Feature List" class="MCListbox (strict)"() -> ("Value"=w440:i32)  [unwired: 2 in, 2 out]
        n203 = property on="Program step" class="LstBox (strict)"() -> ("Value"=w439:i32)  [unwired: 2 in, 2 out]
        n204 = Select(t="STM", s="Motor", f="N") -> (s? t:f=w451:string)
        n205 = call "STM-program.vi"() -> ("OutDir"=w450:i32, "Out Speed"=w448:i32, "Out Degree"=w449:dbl, "Channels (A:B:C:D...) (Out)"=w428:string)  [unwired: 7 in, 1 out]
        n206 = Increment(x=w439) -> (x+1=w434:i32)
        n207 = Bundle By Name(cluster=w446, "Channel Type"=w451, "Channels"=w428, "Wait/Poll (ms)"=u32 0, "Parameter"=u8 0, "STM-Degree"=w449, "STM-Speed"=w448, "Direction"=w450) -> (w431:T20)
        n208 = Index Array(array=w441, index=w440) -> (element=w444:T21)
        n209 = Unbundle By Name(w444) -> ("Steps"=w445:T22)
        n210 = Insert Into Array(array=w445, index=w434, new element=w431) -> (w442:T22)
        n211 = Bundle By Name(cluster=w444, "Steps"=w442) -> (w443:T21)
        n212 = local write "Motor"(FALSE ("Motor")) -> ()
        n213 = call "BuildStepListFromSteps.vi"("Steps"=w442, "Control Channels"=w438, "Feedback Channels"=w437, "AI"=w436) -> ("Step List"=w432:string[])  [unwired: 11 in]
        n214 = Replace Array Subset(array=w441, new element=w443, index=w440) -> (w433:T4)
        n215 = property on="Program step" class="LstBox (strict)"("Key Focus"=TRUE, "Value"=w434, "Item Names"=w432) -> ()  [unwired: 2 in, 2 out]
      }
      event Value Change {
        n216 = event-data() -> ()  [unwired: 1 in, 1 out]
        n217 = property on="Feature List" class="MCListbox (strict)"() -> ("Value"=w454:i32)  [unwired: 2 in, 2 out]
        n218 = Index Array(array=w462, index=w454) -> (element=w465:T21)
        n219 = Bundle By Name(cluster=w471, "Channel Type"="N", "Wait/Poll (ms)"="Wait Time") -> (w467:T20)
        n220 = Unbundle By Name(w465) -> ("Steps"=w466:T22)
        n221 = property on="Program step" class="LstBox (strict)"() -> ("Value"=w468:i32)  [unwired: 2 in, 2 out]
        n222 = Increment(x=w468) -> (x+1=w455:i32)
        n223 = Insert Into Array(array=w466, index=w455, new element=w467) -> (w463:T22)
        n224 = Bundle By Name(cluster=w465, "Steps"=w463) -> (w464:T21)
        n225 = call "BuildStepListFromSteps.vi"("Steps"=w463, "Control Channels"=w460, "Feedback Channels"=w459, "AI"=w457) -> ("Step List"=w458:string[])  [unwired: 11 in]
        n226 = property on="Program step" class="LstBox (strict)"("Item Names"=w458, "Value"=w455, "Key Focus"=TRUE) -> ()  [unwired: 2 in, 2 out]
        n227 = Replace Array Subset(array=w462, new element=w464, index=w454) -> (w461:T4)
      }
      event Value Change {
        n228 = event-data() -> ()  [unwired: 1 in, 2 out]
        n229 = property on="Feature List" class="MCListbox (strict)"() -> ("Value"=w473:i32)  [unwired: 2 in, 2 out]
        n230 = Index Array(array=w484, index=w473) -> (element=w490:T21)
        n231 = property on="Program step" class="LstBox (strict)"() -> ("Value"=w472:i32)  [unwired: 2 in, 2 out]
        n232 = Unbundle By Name(w490) -> ("Item Name"=w488:string, "Item Status"=w487:bool, "Steps"=w486:T22)
        n233 = Equal?(x=w472, y=-1) -> (x = y?=w476:bool)
        n234 = Select(t=0 ("y"), s=w476, f=w472) -> (s? t:f=w474:i32)
        n235 = Delete From Array(array=w486, length=1, index=w474) -> (array with subset deleted=w482:T22)  [unwired: 1 out]
        n236 = Bundle("Item Name"=w488, "Item Status"=w487, "Steps"=w482) -> (w485:T21)  [unwired: 1 in]
        n237 = call "BuildStepListFromSteps.vi"("Steps"=w482, "Control Channels"=w480, "Feedback Channels"=w479) -> ("Step List"=w478:string[])  [unwired: 12 in]
        n238 = Replace Array Subset(array=w484, new element=w485, index=w473) -> (w483:T4)
        n239 = property on="Program step" class="LstBox (strict)"("Item Names"=w478, "Value"=w474, "Key Focus"=TRUE) -> ()  [unwired: 2 in, 2 out]
      }
      event Value Change {
        n240 = event-data() -> ()  [unwired: 1 in, 1 out]
        n241 = for {
          tunnel: w493 -> [w540] mode=indexing
          tunnel: [w535] -> w501 mode=indexing
          shift-right: [w534] -> w502
          shift-left: w509 -> [w537]
          n242 = Unbundle By Name(w540) -> ("Steps"=w541:T22, "Item Name"=w539:string, "Item Status"=w538:bool)
          n243 = Array Size(array=w541) -> (size(s)=w536:i32)
          n244 = case shown="Default" w536 {
            tunnel: w541 -> [_ w548]
            tunnel: w539 -> [_ w550]
            tunnel: w538 -> [_ w549]
            tunnel: [w543 w546] -> w534
            tunnel: w537 -> [w543 w544]
            tunnel: [FALSE TRUE] -> w535
            frame 0 {
            }
            frame Default {
              n245 = Bundle("Item Name"=w550, "Item Status"=w549, "Steps"=w548) -> (w545:T21)  [unwired: 1 in]
              n246 = Build Array (concatenate)(w544, w545) -> (w546:T4)
            }
          }
        }
        n247 = And Array Elements(Boolean array=w501) -> (logical AND=w500:bool)
        n248 = case shown="True" w500 {
          tunnel: [w513 w515] -> w495
          tunnel: w494 -> [_ w523]
          tunnel: [_ w521] -> w503
          tunnel: w502 -> [_ w516]
          tunnel: enum16{"Read", "Write"}."Write" ("Read/Write") -> [_ w522]
          tunnel: "Feature List successfully saved." -> [_ w520]
          tunnel: "Error in saving Feature List." -> [_ w519]
          tunnel: "Can't save Feature List as at least one feature doesn't have steps.\nPlease check." ("message") -> [w514 w518]
          tunnel: w493 -> [w513 _]
          frame False {
            n249 = One Button Dialog(message=w514) -> ()  [unwired: 1 in, 1 out]
          }
          frame True {
            n250 = call "FileIO-ReadWrite-FeatureList.vi"("Filepath"=w523, "Feature List (In)"=w516, "Read/Write"=w522) -> ("Feature List (Out)"=w515:T4, "Error Out"=w521:errorcluster)  [unwired: 11 in]
            n251 = case shown="Error" w521 {
              tunnel: w520 -> [w524 _]
              tunnel: w519 -> [_ w525]
              tunnel: w518 -> [_ _]
              tunnel: [w524 w525] -> w517
              frame No Error {
              }
              frame Error {
              }
            }
            n252 = One Button Dialog(message=w517) -> ()  [unwired: 1 in, 1 out]
          }
        }
        n253 = disable-structure shown="Enabled" {
          frame Disabled {
            n254 = call "Program seq path.vi"() -> ()  [unwired: 11 in, 1 out]
          }
          frame Enabled {
          }
        }
        n255 = Index Array(array=w495, index=0) -> (element=w507:T21)
        n256 = Unbundle By Name(w507) -> ("Steps"=w506:T22)
        n257 = for {
          tunnel: [w532] -> w492 mode=indexing
          tunnel: w495 -> [w527] mode=indexing
          tunnel: [w526] -> _
          i -> [w526]
          n258 = Unbundle By Name(w527) -> ("Item Name"=w533:string, "Item Status"=w531:bool)
          n259 = Select(t="Active", s=w531, f="Inactive") -> (s? t:f=w528:string)
          n260 = Build Array(w533, w528) -> (w532:string[])
        }
        n261 = call "BuildStepListFromSteps.vi"("Steps"=w506, "Control Channels"=w512, "Feedback Channels"=w511, "AI"=w504) -> ("Step List"=w510:string[])  [unwired: 11 in]
        n262 = property on="Program step" class="LstBox (strict)"("Item Names"=w510, "Value"=0 ("Step feautre list")) -> ()  [unwired: 2 in, 2 out]
        n263 = property on="Feature List" class="MCListbox (strict)"("ItemNames"=w492, "Value"=0 ("Feautre list")) -> ()  [unwired: 2 in, 2 out]
      }
      event Value Change {
        n264 = event-data() -> ()  [unwired: 1 in, 1 out]
      }
      event "Program step": Double Click {
        n265 = event-data() -> ("Row"=w567:i32)  [unwired: 1 in, 8 out]
        n266 = property on="Program step" class="LstBox (strict)"() -> ("Item Names"=w568:string[])  [unwired: 2 in, 2 out]
        n267 = Index Array(array=w568, index=w567) -> (element=w558:string)
        n268 = String Length(string=w558) -> (length=w557:i32)
        n269 = String Subset(string=w558, length (rest)=2 ("length (rest)")) -> (substring=w563:string)  [unwired: 1 in]
        n270 = String Subset(string=w558, length (rest)=4 ("length (rest)")) -> (substring=w561:string)  [unwired: 1 in]
        n271 = Less Or Equal?(x=w557, y=0) -> (x <= y?=w554:bool)
        "x <= y?" <- w554
        n272 = Equal?(x=w561, y="Wait") -> (x = y?=w559:bool)
        n273 = Equal?(x=w563, y="Ch") -> (x = y?=w564:bool)
        n274 = case shown="False" w554 {
          tunnel: w576 -> [w587 _]
          tunnel: w575 -> [w586 w650]
          tunnel: w574 -> [w585 _]
          tunnel: w573 -> [w584 _]
          tunnel: w572 -> [w583 _]
          tunnel: [w582 w650] -> w571
          tunnel: [w581 w651] -> w570
          tunnel: w569 -> [w580 w651]
          tunnel: w564 -> [w579 _]
          tunnel: w559 -> [w578 _]
          tunnel: enum32{"Output", "Input"}."Output" ("y") -> [w577 _]
          frame False {
            n275 = case shown="False" w578 {
              tunnel: w587 -> [w604 w637]
              tunnel: w586 -> [w603 w636]
              tunnel: w585 -> [w602 w640]
              tunnel: w584 -> [w601 w639]
              tunnel: w583 -> [w600 w638]
              tunnel: [w599 w635] -> w582
              tunnel: [w598 w634] -> w581
              tunnel: w580 -> [w592 _]
              tunnel: w579 -> [w591 _]
              tunnel: w577 -> [w589 _]
              frame False {
                n276 = call "DO Control.vi"("s"=w591) -> ("Feedback"=w594:i32[], "Parameter (Out)"=w595:u8, "Control Channel"=w597:i32[], "Poll Time (Out)"=w596:u32, "Tab Control 2"=w588:enum32{"Output", "Input"}, "Cancel"=w590:bool)  [unwired: 5 in]
                n277 = Equal?(x=w588, y=w589) -> (x = y?=w593:bool)
                n278 = case shown="False" w590 {
                  tunnel: w604 -> [w629 _]
                  tunnel: w603 -> [w628 w631]
                  tunnel: w602 -> [w627 _]
                  tunnel: w601 -> [w626 _]
                  tunnel: w600 -> [w625 _]
                  tunnel: [w624 w631] -> w599
                  tunnel: [w623 w632] -> w598
                  tunnel: w597 -> [w614 _]
                  tunnel: w596 -> [w613 _]
                  tunnel: w595 -> [w612 _]
                  tunnel: w594 -> [w611 _]
                  tunnel: w593 -> [w605 _]
                  tunnel: w592 -> [_ w632]
                  frame False {
                    n279 = property on="Feature List" class="MCListbox (strict)"() -> ("Value"=w615:i32)  [unwired: 2 in, 2 out]
                    n280 = Index Array(array=w628, index=w615) -> (element=w620:T21)
                    n281 = Select(t="C", s=w605, f="F") -> (s? t:f=w608:string)
                    n282 = Select(t=w614, s=w605, f=w611) -> (s? t:f=w607:i32[])
                    n283 = disable-structure shown="Disabled" {
                      disable-tunnel: w605 -> [w630 _]
                      frame Disabled {
                        n284 = call "Configuration-PromptForChannelParameters_timer.vi"("Control/Feedback\n(Default: False = Feedback)"=w630) -> ()  [unwired: 13 in, 2 out]
                      }
                      frame Enabled {
                      }
                    }
                    n285 = call "ConvertNumericChannelsToStringChannels.vi"("Channels (In)"=w607) -> ("Channels (A:B:C:D...) (Out)"=w606:string)  [unwired: 14 in]
                    n286 = Unbundle By Name(w620) -> ("Steps"=w622:T22)
                    n287 = Bundle By Name(cluster=w629, "Channel Type"=w608, "Channels"=w606, "Wait/Poll (ms)"=w613, "Parameter"=w612) -> (w621:T20)
                    n288 = property on="Program step" class="LstBox (strict)"() -> ("Value"=w616:i32)  [unwired: 2 in, 2 out]
                    n289 = Replace Array Subset(array=w622, new element=w621, index=w616) -> (w618:T22)
                    n290 = Bundle By Name(cluster=w620, "Steps"=w618) -> (w619:T21)
                    n291 = call "BuildStepListFromSteps.vi"("Steps"=w618, "Control Channels"=w625, "Feedback Channels"=w626, "AI"=w627) -> ("Step List"=w623:string[])  [unwired: 11 in]
                    "Step List 2" <- w623
                    n292 = Replace Array Subset(array=w628, new element=w619, index=w615) -> (w624:T4)
                    n293 = property on="Program step" class="LstBox (strict)"("Key Focus"=TRUE, "Value"=w616, "Item Names"=w623) -> ()  [unwired: 2 in, 2 out]
                  }
                  frame True {
                  }
                }
              }
              frame True {
                n294 = property on="Feature List" class="MCListbox (strict)"() -> ("Value"=w641:i32)  [unwired: 2 in, 2 out]
                n295 = call "Timer.vi"() -> ("Wait Time out"=w633:u32)  [unwired: 10 in, 1 out]
                n296 = Index Array(array=w636, index=w641) -> (element=w645:T21)
                n297 = Bundle By Name(cluster=w637, "Channel Type"="N", "Wait/Poll (ms)"=w633) -> (w647:T20)
                n298 = Unbundle By Name(w645) -> ("Steps"=w646:T22)
                n299 = property on="Program step" class="LstBox (strict)"() -> ("Value"=w648:i32)  [unwired: 2 in, 2 out]
                n300 = Replace Array Subset(array=w646, new element=w647, index=w648) -> (w643:T22)
                n301 = Bundle By Name(cluster=w645, "Steps"=w643) -> (w644:T21)
                n302 = call "BuildStepListFromSteps.vi"("Steps"=w643, "Control Channels"=w638, "Feedback Channels"=w639, "AI"=w640) -> ("Step List"=w634:string[])  [unwired: 11 in]
                n303 = property on="Program step" class="LstBox (strict)"("Item Names"=w634, "Value"=w648, "Key Focus"=TRUE) -> ()  [unwired: 2 in, 2 out]
                n304 = Replace Array Subset(array=w636, new element=w644, index=w641) -> (w635:T4)
              }
            }
          }
          frame True {
          }
        }
      }
      event Panel Close? {
        n305 = event-data() -> ()  [unwired: 1 in, 1 out]
        n306 = event-data("Discard?"=TRUE) -> ()  [unwired: 1 in, 1 out]
      }
    }
  }
  "Error Out" <- w23
